vi "fpga.orderbook.test.harness.vi"   [LabVIEW 2020]
uses:
  <vilib>/Platform/TimedLoop/XDataNode/timing_clust.ctl
  <vilib>/Platform/TimedLoop/XDataNode/nitl_modes.ctl
  <vilib>/Platform/TimedLoop/XDataNode/wakeup.ctl
  Test/test.data.in.ctl
  <vilib>/rvi/DataTransferAndStorage/Container/Common/niFpgaContainerGetUniqueNameForEmu.vi
  <vilib>/rvi/DataTransferAndStorage/Container/Common/niFpgaContainerSetEmuInfo.vi
  <vilib>/rvi/eio/common/nirviEmuReportErrorAndStop.vi
  <vilib>/rvi/Emulation/niFpgaSctlEmulationGetInTimedLoop.vi
  <vilib>/rvi/Emulation/niFpgaEmulationReportErrorSimple.vi
  <vilib>/rvi/Emulation/niFpgaGetClockAttributes.vi
  <vilib>/rvi/Emulation/niFpgaCriticalErrorInLSC.vi
  <vilib>/rvi/interface/RandomDataEmulation/niFpgaRandomDataHandleErrors.vi
  <vilib>/rvi/DataTransferAndStorage/Container/Common/niFpgaContainerExecOnDevCompGetState.vi
  <vilib>/rvi/Emulation/niFpgaEmulationIsFPGAContextNoSignature.vi
  <vilib>/rvi/errors/niFpgaSetErrorForExecOnDevCompSimple.vi
  <vilib>/rvi/FIFO/Fifo_Resource/nirvififoEmulationSetSize.vi
  <vilib>/rvi/FIFO/Fifo_Resource/nirviFifoEmulationQueueMgr.vi
  <instcachedir>/0/nirviFifoEmulationQueueMgr_E5CAEC123FF24DC58D834DCA3CDAA9B5.lvgen/nirviFifoEmulationQueueMgr_E5CAEC123FF24DC58D834DCA3CDAA9B5_015.vi
  <vilib>/rvi/FIFO/Fifo_Resource/nirvififoEmulationDetermineInputValidOut.vi
  <vilib>/rvi/FIFO/Fifo_Resource/nirvififoEmulationCreateLock.vi
  <vilib>/rvi/Emulation/niFpgaProcessEmulError.vi
  <vilib>/rvi/FIFO/Fifo_Resource/nirvififoEmulationObtainLock.vi
  <vilib>/rvi/FIFO/Fifo_Resource/nirvififoEmulationReleaseLock.vi
  <vilib>/rvi/occurrence/nirviWaitOnOccurrenceBase.vi
  <vilib>/rvi/errors/nirviReportUnexpectedCaseInternalError.vi
  <vilib>/rvi/errors/nirviReportUnexpectedCaseInternalError (U32).vi
  <vilib>/Utility/error.llb/Clear Errors.vi
  <instcachedir>/0/nirviFifoEmulationQueueMgr_E5CAEC123FF24DC58D834DCA3CDAA9B5.lvgen/nirviFifoEmulationQueueMgr_E5CAEC123FF24DC58D834DCA3CDAA9B5_002.vi
  <vilib>/Platform/TimedLoop/XDataNode/XDataNode.xnode
  <vilib>/rvi/LocalResourceManager/LocalResourceManager.xnode
  <vilib>/rvi/DataTransferAndStorage/Container/XNode/niFpgaContainer.xnode
  <vilib>/rvi/interface/RandomDataEmulation/nirviRandomDataFpgaReadWriteTemplate.vi
  <vilib>/rvi/FIFO/Fifo_Resource/niFpgaFifoEmulationRefIn.vi
  <vilib>/Platform/TimedLoop/XDataNode/XDNodeRunTimeDep.lvlib
types:
  T1 = typedef "XDNodeRunTimeDep.lvlib/timing_clust.ctl" = cluster{"Expected End [f-1]":u64, "Actual End [f-1]":u64, "Finished Late? [f-1]":bool, "Expected End [i-1]":u64, "Actual End [i-1]":u64, "Finished Late? [i-1]":bool, "Expected Start [i]":u64, "Actual Start [i]":u64, "Expected Start [f]":u64, "Actual Start [f]":u64, "Source Name":string, "Structure Name":string, "Period":i64, "Deadline":i64, "Offset":i64, "Start":i64, "Priority":i32, "Timeout":i32, "Mode":T2, "Wakeup Reason":T3, "Error":errorcluster, "Source Type":string, "Secondary Source Type":string, "Global End Time":u64, "Global Start Time":u64, "Frame Duration":u64, "Iteration Duration":u64, "Assigned CPU":i32, "I/O Scan Engine Mode":u32}
  T2 = typedef "XDNodeRunTimeDep.lvlib/nitl_modes.ctl" = enum32{"No Change", "Process missed periods, maintain original phase", "Discard missed periods, maintain original phase", "Process missed periods, ignore original phase", "Discard missed periods, ignore original phase"}
  T3 = typedef "XDNodeRunTimeDep.lvlib/wakeup.ctl" = enum32{"Normal", "Aborted", "Asynchronous wakeup", "Timing source error", "Timed loop error", "Timeout"}
  T4 = typedef "test.data.in.ctl" = cluster{"data":u8, "end_of_frame":bool}
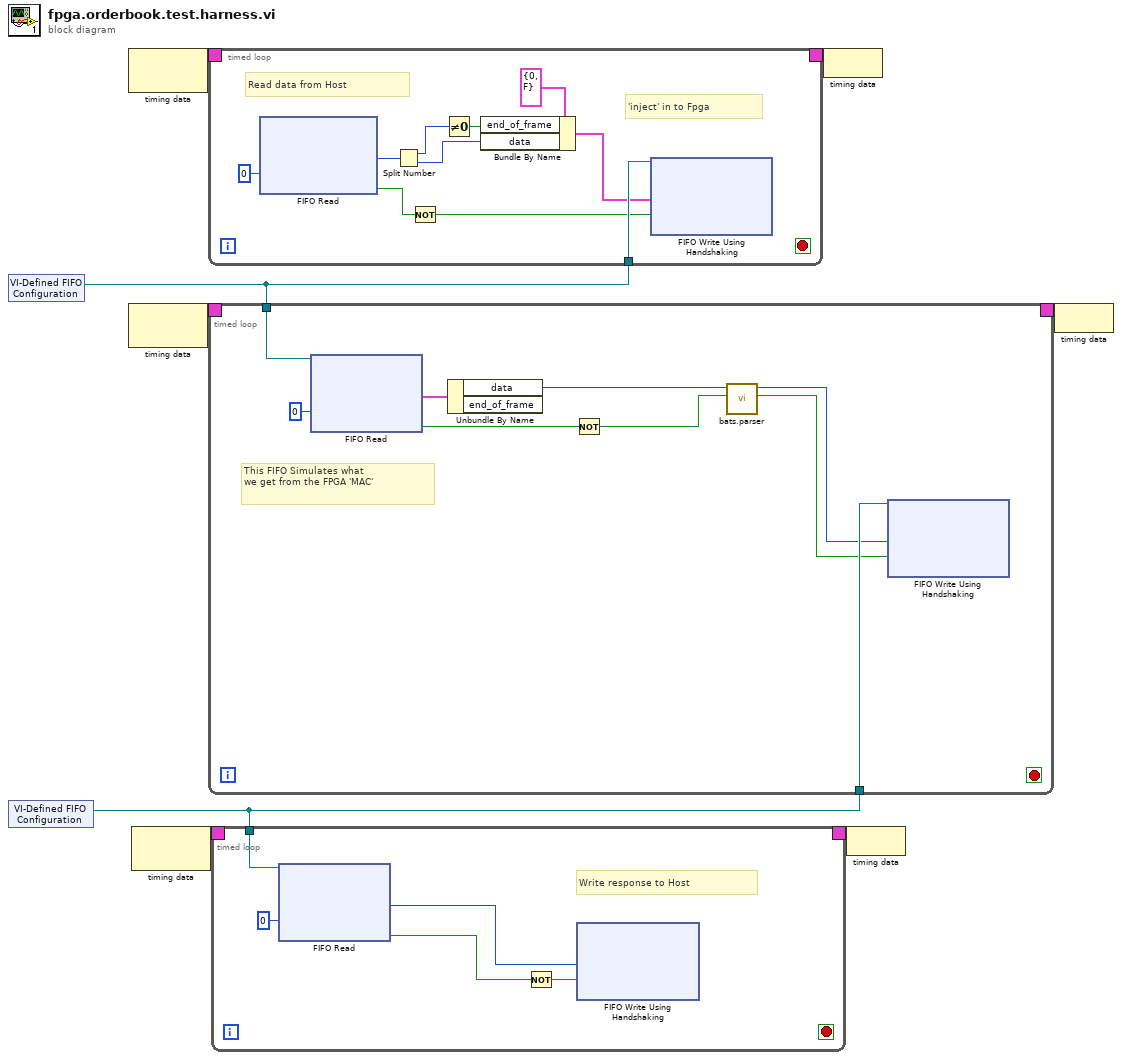
[diagram p0: block diagram]
diagram:
  n1 = xnode "VI-Defined FIFO Configuration"() -> ("FIFO Out"=w4:refnum<k21>)
  n2 = xnode "VI-Defined FIFO Configuration"() -> ("FIFO Out"=w1:refnum<k21>)
  n3 = node-c288() -> (w8:T1)  [unwired: 1 in]
  n4 = node-c288() -> (w6:T1)  [unwired: 1 in]
  n5 = node-c288() -> (w3:T1)  [unwired: 1 in]
  n6 = timed-loop {
    timing: w8 -> [_]
    timing-out: [_] -> w7
    tunnel: w4 -> [w18]
    stop <- _ stop-if-true
    # "'inject' in to Fpga"
    # "Read data from Host"
    n7 = xnode "FIFO Read"("Timeout"=0) -> ("Element"=w14:u16, "Timed Out?"=w16:bool)  [unwired: 1 in, 1 out]
    n8 = Split Number(x=w14) -> (hi(x)=w10:u8, lo(x)=w12:u8)
    n9 = Not(x=w16) -> (.not. x?=w15:bool)
    n10 = Not Equal To 0?(x=w10) -> (x != 0?=w11:bool)
    n11 = Bundle By Name(cluster=T4 {"data"=0, "end_of_frame"=FALSE} ("Cluster"), "end_of_frame"=w11, "data"=w12) -> (w9:T4)
    n12 = xnode "FIFO Write Using Handshaking"("Element"=w9, "Input Valid"=w15, "FIFO In"=w18) -> ()  [unwired: 2 out]
  }
  n13 = timed-loop {
    timing: w6 -> [_]
    timing-out: [_] -> w5
    tunnel: w4 -> [w29]
    tunnel: w1 -> [w25]
    stop <- _ stop-if-true
    # "This FIFO Simulates what\nwe get from the FPGA 'MAC'"
    n14 = xnode "FIFO Read"("Timeout"=0, "FIFO In"=w29) -> ("Element"=w27:cluster{"data":u8, "end_of_frame":bool}, "Timed Out?"=w26:bool)  [unwired: 1 out]
    n15 = Unbundle By Name(w27) -> ("data"=w21:u8)  [unwired: 1 out]
    n16 = Not(x=w26) -> (.not. x?=w22:bool)
    n17 = call "bats.parser.vi"("data_valid"=w22, "data"=w21) -> ("tvalid"=w24:bool, "tdata"=w23:u8)  [unwired: 7 in, 1 out]
    n18 = xnode "FIFO Write Using Handshaking"("Element"=w23, "Input Valid"=w24, "FIFO In"=w25) -> ()  [unwired: 2 out]
  }
  n19 = timed-loop {
    timing: w3 -> [_]
    timing-out: [_] -> w2
    tunnel: w1 -> [w36]
    stop <- _ stop-if-true
    # "Write response to Host"
    n20 = xnode "FIFO Read"("Timeout"=0, "FIFO In"=w36) -> ("Element"=w32:u8, "Timed Out?"=w34:bool)  [unwired: 1 out]
    n21 = Not(x=w34) -> (.not. x?=w33:bool)
    n22 = xnode "FIFO Write Using Handshaking"("Element"=w32, "Input Valid"=w33) -> ()  [unwired: 1 in, 2 out]
  }
  n23 = node-c288(w7) -> ()
  n24 = node-c288(w2) -> ()
  n25 = node-c288(w5) -> ()
